vi "SaveConfig.vi"(8 "error in (no error)":errorcluster, 10 "config file path (Empty: use configured)":path, 11 "BASE in":refnum<class "BASE.lvclass">) -> (0 "error out":errorcluster, 3 "BASE out":refnum<class "BASE.lvclass">)   [LabVIEW 2019, in "BASE.lvlib" / "BASE.lvclass"]
uses:
  BASE.lvclass
  BASE.lvclass/BASE.ctl
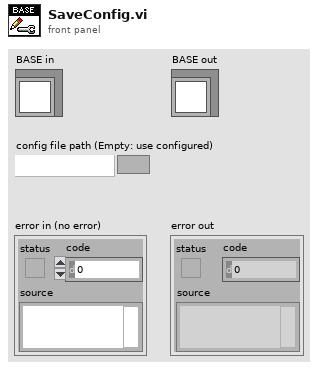
[diagram p1: front panel]
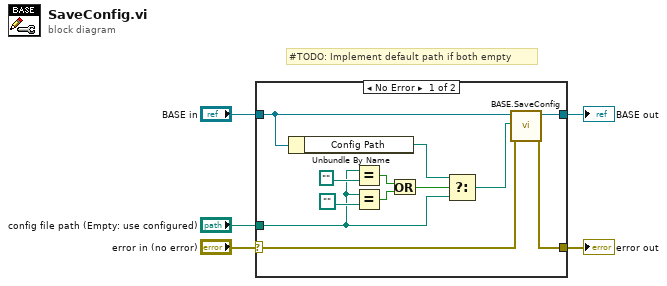
[diagram p0: block diagram]
diagram:
  # "#TODO: Implement default path if both empty"
  n1 = case shown="No Error" "error in (no error)" {
    selector: "error in (no error)" -> [w6 w18]
    tunnel: [w17 w19] -> w5
    tunnel: [w16 w18] -> w4
    tunnel: "config file path (Empty: use configured)" -> [w10 _]
    tunnel: "BASE in" -> [w8 w19]
    frame No Error {
      n2 = Unbundle By Name(w8) -> ("Config Path"=w9:path)
      n3 = Equal?(x=w10, y=path "") -> (x = y?=w12:bool)
      n4 = Equal?(x=w10, y=path "") -> (x = y?=w13:bool)
      n5 = Or(x=w12, y=w13) -> (x .or. y?=w11:bool)
      n6 = Select(t=w9, s=w11, f=w10) -> (s? t:f=w7:path)
      n7 = call-dynamic "BASE.SaveConfig.vi"("error in (no error)"=w6, "config file path"=w7, "BASE in"=w8) -> ("error out"=w16:errorcluster, "BASE out"=w17:refnum<class "BASE.lvclass">)  [unwired: 7 in]
    }
    frame Error {
    }
  }
  "error out" <- w4
  "BASE out" <- w5
